vi "Read Folder Index.vi"(8 "error in (no error)":errorcluster, 11 "File or Folder Path":path) -> (0 "error out":errorcluster, 3 "Files":path[](array[path]))   [LabVIEW 2016, in "LVtoITX.lvclass"]
uses:
  LVtoITX.lvclass
  <vilib>/Utility/file.llb/Read Delimited Spreadsheet (string).vi
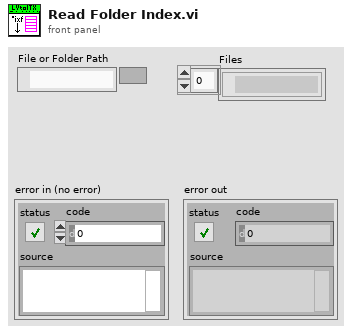
[diagram p1: front panel]
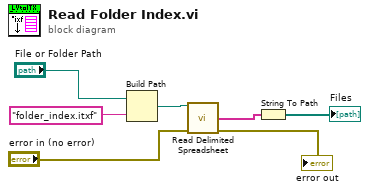
[diagram p0: block diagram]
diagram:
  n1 = Build Path(base path="File or Folder Path", name or relative path="folder_index.itxf") -> (appended path=w6:path)
  n2 = call-poly <vilib>:"Read Delimited Spreadsheet.vi"("file path (dialog if empty)"=w6, "error in (no error)"="error in (no error)") -> ("first row"=w1:string[], "error out"=→"error out":errorcluster)  [unwired: 8 in, 4 out]
  n3 = String To Path(string=w1) -> (path=→"Files":path[])
